vi "MoveZ.vi"(2 "RetPos":bool, 3 "Wait":bool=TRUE, 4 "GoTo (mm)":sgl, 5 "MG17Motor":refnum<k7>(container)) -> (0 "StartPosition(um)":sgl, 1 "EndPosition (um)":sgl)   [LabVIEW 2015]
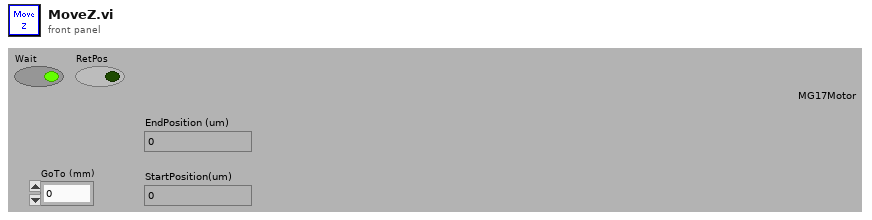
[diagram p1: front panel]
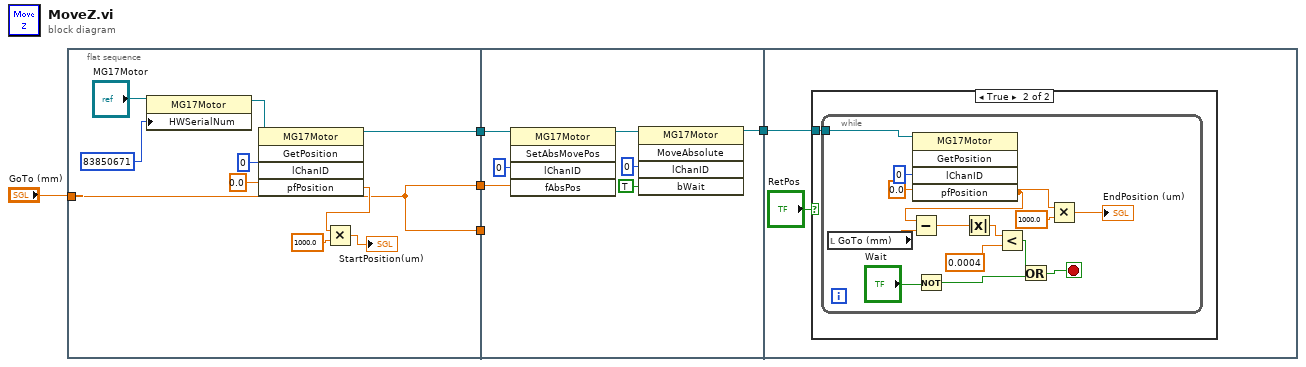
[diagram p0: block diagram]
diagram:
  n1 = flat-sequence {
    tunnel: [w14] -> w5
    tunnel: [w9] -> w4
    tunnel: [w9] -> w3
    tunnel: "GoTo (mm)" -> [w9]
    tunnel: w5 -> [w22]
    tunnel: w4 -> [w20]
    tunnel: w3 -> [_]
    tunnel: [w16] -> w2
    tunnel: w2 -> [w24]
    frame #0 {
      n2 = property class="MG17Motor"(reference="MG17Motor", "HWSerialNum"=83850671) -> (reference out=w7:refnum<k7>)  [unwired: 1 in, 1 out]
      n3 = invoke class="MG17Motor" method="GetPosition"(reference=w7, "lChanID"=0, "pfPosition"=sgl 0.0) -> (reference out=w14:refnum<k7>, "pfPosition"=w12:sgl)  [unwired: 2 in, 3 out]
      n4 = Multiply(x=w12, y=sgl 1000.0) -> (x*y=→"StartPosition(um)":sgl)
    }
    frame #1 {
      n5 = invoke class="MG17Motor" method="SetAbsMovePos"(reference=w22, "lChanID"=0, "fAbsPos"=w20) -> (reference out=w21:refnum<k7>)  [unwired: 2 in, 4 out]
      n6 = invoke class="MG17Motor" method="MoveAbsolute"(reference=w21, "lChanID"=0, "bWait"=TRUE) -> (reference out=w16:refnum<k7>)  [unwired: 2 in, 4 out]
    }
    frame #2 {
      n7 = case shown="True" "RetPos" {
        tunnel: w24 -> [_ w25]
        frame False {
        }
        frame True {
          n8 = while {
            tunnel: w25 -> [w34]
            stop <- w26 stop-if-true
            n9 = local read "GoTo (mm)"() -> (w30:sgl)
            n10 = invoke class="MG17Motor" method="GetPosition"(reference=w34, "lChanID"=0, "pfPosition"=sgl 0.0) -> ("pfPosition"=w32:sgl)  [unwired: 2 in, 4 out]
            n11 = Subtract(x=w32, y=w30) -> (x-y=w37:sgl)
            n12 = Not(x="Wait") -> (.not. x?=w28:bool)
            n13 = Absolute Value(x=w37) -> (abs(x)=w36:sgl)
            n14 = Less?(x=w36, y=0.0004) -> (x < y?=w27:bool)
            n15 = Or(x=w27, y=w28) -> (x .or. y?=w26:bool)
            n16 = Multiply(x=w32, y=sgl 1000.0) -> (x*y=→"EndPosition (um)":sgl)
          }
        }
      }
    }
  }
